vi "example_write.vi"(6 "dvr":refnum<data-value>, 8 "error in (no error)":errorcluster, 10 "y_axis":dbl[](array[numeric]), 11 "x_axis":dbl) -> (0 "error out":errorcluster, 3 "index":i32)   [LabVIEW 2015, in "lv-graph.lvlib"]
uses:
  lv-graph.lvlib
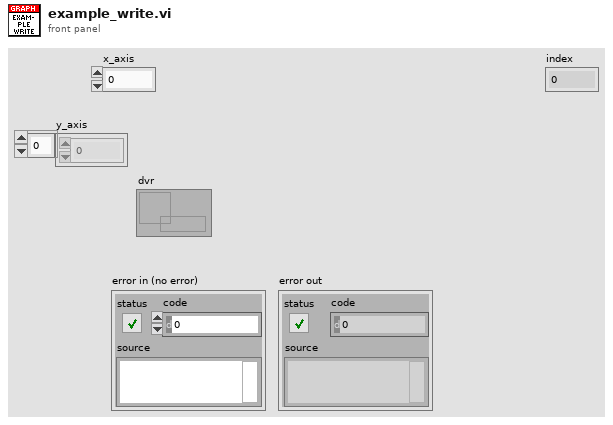
[diagram p1: front panel]
types:
  T1 = cluster{"index":i32, "x_axis":dbl[], "y_axis":dbl[][]}
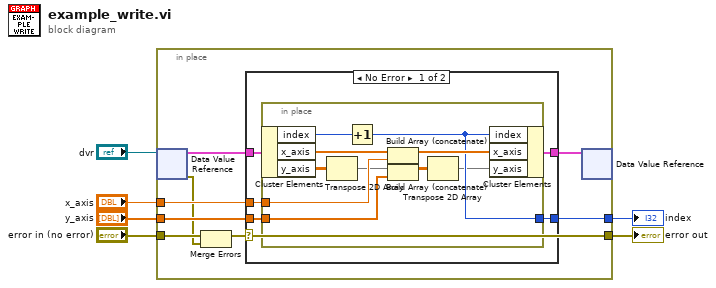
[diagram p0: block diagram]
diagram:
  n1 = in-place {
    in-place-border: "x_axis" -> [w14]
    in-place-border: "y_axis" -> [w13]
    in-place-border: "error in (no error)" -> [w10]
    in-place-border: [w8] -> w2
    in-place-border: [w7] -> w1
    n2 = in-place-dvr #1("dvr") -> (w11:T1, w9:errorcluster)
    n3 = Merge Errors(w10, w9) -> (w8:errorcluster)
    n4 = case shown="No Error" w8 {
      tunnel: w14 -> [w19 _]
      tunnel: w13 -> [w18 _]
      tunnel: [w17 w30] -> w12
      tunnel: w11 -> [w16 w30]
      tunnel: [w15 _] -> w7
      frame No Error {
        n5 = in-place {
          in-place-border: w19 -> [w29]
          in-place-border: w18 -> [w28]
          in-place-border: [w24] -> w15
          n6 = in-place-cluster #2(w16) -> ("index"=w27:i32, "x_axis"=w23:dbl[], "y_axis"=w22:dbl[][])
          n7 = Transpose 2D Array(2D array=w22) -> (transposed array=w21:dbl[][])
          n8 = Increment(x=w27) -> (x+1=w24:i32)
          n9 = Build Array (concatenate)(w23, w29) -> (w26:dbl[])
          n10 = Build Array (concatenate)(w21, w28) -> (w25:dbl[][])
          n11 = Transpose 2D Array(2D array=w25) -> (transposed array=w20:dbl[][])
          n12 = in-place-cluster #2("index"=w24, "x_axis"=w26, "y_axis"=w20) -> (w17:T1)
        }
      }
      frame Error {
      }
    }
    n13 = in-place-dvr #1(w12) -> ()  [unwired: 2 out]
  }
  "error out" <- w2
  "index" <- w1
